vi "test_read-nmea-data2.vi"() -> ()   [LabVIEW 2019] (continued)
F9P\t$GBGSV,2,1,06,07,,,23,11,48,133,26,14,87,101,29,28,,,23,1*76\n\t\n15:15:02.67\tF9P\t$GBGSV,2,2,06,33,62,220,31,34,,,25,1*46\n\t\n15:15:02.69\tF9P\t$GBGSV,1,1,03,11,48,133,,14,87,101,28,33,62,220,,3*4E\n\t\n15:15:02.71\tF9P\t$GNGLL,3723.60146,N,12656.95282,E,061504.00,A,A*73\n\t\n15:15:02.73\tF9P\t\t\n15:15:02.75\tF9P\t\t\n15:15:02.77\tF9P\t\t\n15:15:02.79\tF9P\t\t\n15:15:02.81\tF9P\t\t\n15:15:02.83\tF9P\t\t\n15:15:02.85\tF9P\t\t\n15:15:02.87\tF9P\t\t\n15:15:02.89\tF9P\t\t\n15:15:02.91\tF9P\t\t\n15:15:02.93\tF9P\t\t\n15:15:02.95\tF9P\t\t\n15:15:02.97\tF9P\t\t\n15:15:02.99\tF9P\t\t\n15:15:03.02\tF9P\t\t\n15:15:03.04\tF9P\t\t\n15:15:03.06\tF9P\t\t\n15:15:03.08\tF9P\t\t\n15:15:03.10\tF9P\t\t\n15:15:03.12\tF9P\t\t\n15:15:03.14\tF9P\t\t\n15:15:03.16\tF9P\t\t\n15:15:03.18\tF9P\t\t\n15:15:03.20\tF9P\t\t\n15:15:03.22\tF9P\t\t\n15:15:03.24\tF9P\t$GNRMC,061505.00,A,3723.60131,N,12656.95173,E,2.899,253.95,250720,,,A,V*02\n\t\n15:15:03.26\tF9P\t$GNVTG,253.95,T,,M,2.899,N,5.368,K,A*29\n\t\n15:15:03.28\tF9P\t$GNGGA,061505.00,3723.60131,N,12656.95173,E,1,12,0.74,45.5,M,18.5,M,,*72\n\t\n15:15:03.30\tF9P\t$GNGSA,A,3,12,06,19,05,17,09,04,02,,,,,1.25,0.74,1.01,1*05\n\t\n15:15:03.32\tF9P\t$GNGSA,A,3,85,70,71,84,,,,,,,,,1.25,0.74,1.01,2*07\n\t\n15:15:03.34\tF9P\t$GNGSA,A,3,36,19,11,04,09,12,,,,,,,1.25,0.74,1.01,3*05\n\t\n15:15:03.36\tF9P\t$GNGSA,A,3,14,11,33,,,,,,,,,,1.25,0.74,1.01,4*04\n\t\n15:15:03.38\tF9P\t$GPGSV,3,1,09,02,56,320,26,04,17,043,37,05,38,248,39,06,64,051,39,1*6A\n\t\n15:15:03.40\tF9P\t$GPGSV,3,2,09,09,44,072,38,12,23,275,27,17,31,154,31,19,51,157,27,1*60\n\t\n15:15:03.42\tF9P\t$GPGSV,3,3,09,25,12,306,15,1*58\n\t\n15:15:03.44\tF9P\t$GPGSV,3,1,09,02,56,320,,04,17,043,22,05,38,248,27,06,64,051,29,6*63\n\t\n15:15:03.46\tF9P\t$GPGSV,3,2,09,09,44,072,29,12,23,275,18,17,31,154,20,19,51,157,,6*6E\n\t\n15:15:03.48\tF9P\t$GPGSV,3,3,09,25,12,306,,6*5B\n\t\n15:15:03.50\tF9P\t$GLGSV,2,1,08,69,10,031,26,70,70,037,29,71,54,207,35,72,05,210,,1*73\n\t\n15:15:03.52\tF9P\t$GLGSV,2,2,08,77,01,324,,84,19,123,17,85,69,072,25,86,38,331,,1*72\n\t\n15:15:03.54\tF9P\t$GLGSV,2,1,08,69,10,031,18,70,70,037,,71,54,207,25,72,05,210,,3*76\n\t\n15:15:03.56\tF9P\t$GLGSV,2,2,08,77,01,324,,84,19,123,22,85,69,072,27,86,38,331,,3*74\n\t\n15:15:03.58\tF9P\t$GAGSV,2,1,08,02,08,296,10,04,67,115,37,09,33,193,26,11,72,001,24,7*7E\n\t\n15:15:03.60\tF9P\t$GAGSV,2,2,08,12,39,103,31,19,25,045,33,25,08,248,,36,27,309,22,7*77\n\t\n15:15:03.62\tF9P\t$GAGSV,2,1,08,02,08,296,,04,67,115,,09,33,193,,11,72,001,,2*7C\n\t\n15:15:03.64\tF9P\t$GAGSV,2,2,08,12,39,103,,19,25,045,23,25,08,248,,36,27,309,,2*71\n\t\n15:15:03.66\tF9P\t$GBGSV,2,1,06,07,,,21,11,48,133,26,14,87,101,22,28,,,23,1*7F\n\t\n15:15:03.68\tF9P\t$GBGSV,2,2,06,33,62,220,30,34,,,25,1*47\n\t\n15:15:03.70\tF9P\t$GBGSV,1,1,03,11,48,133,,14,87,101,28,33,62,220,,3*4E\n\t\n15:15:03.72\tF9P\t$GNGLL,3723.60131,N,12656.95173,E,061505.00,A,A*7F\n\t\n15:15:03.74\tF9P\t\t\n15:15:03.76\tF9P\t\t\n15:15:03.78\tF9P\t\t\n15:15:03.80\tF9P\t\t\n15:15:03.82\tF9P\t\t\n15:15:03.84\tF9P\t\t\n15:15:03.86\tF9P\t\t\n15:15:03.88\tF9P\t\t\n15:15:03.90\tF9P\t\t\n15:15:03.92\tF9P\t\t\n15:15:03.94\tF9P\t\t\n15:15:03.96\tF9P\t\t\n15:15:03.98\tF9P\t\t\n15:15:04.00\tF9P\t\t\n15:15:04.02\tF9P\t\t\n15:15:04.04\tF9P\t\t\n15:15:04.06\tF9P\t\t\n15:15:04.08\tF9P\t\t\n15:15:04.10\tF9P\t\t\n15:15:04.12\tF9P\t\t\n15:15:04.14\tF9P\t\t\n15:15:04.16\tF9P\t\t\n15:15:04.18\tF9P\t\t\n15:15:04.20\tF9P\t\t\n15:15:04.22\tF9P\t\t\n15:15:04.24\tF9P\t$GNRMC,061506.00,A,3723.60131,N,12656.95050,E,2.846,256.78,250720,,,A,V*05\n\t\n15:15:04.26\tF9P\t$GNVTG,256.78,T,,M,2.846,N,5.272,K,A*27\n\t\n15:15:04.28\tF9P\t$GNGGA,061506.00,3723.60131,N,12656.95050,E,1,12,0.74,45.5,M,18.5,M,,*71\n\t\n15:15:04.30\tF9P\t$GNGSA,A,3,12,06,19,05,17,09,04,02,,,,,1.25,0.74,1.01,1*05\n\t\n15:15:04.32\tF9P\t$GNGSA,A,3,85,70,71,84,,,,,,,,,1.25,0.74,1.01,2*07\n\t\n15:15:04.34\tF9P\t$GNGSA,A,3,36,19,11,04,09,12,,,,,,,1.25,0.74,1.01,3*05\n\t\n15:15:04.36\tF9P\t$GNGSA,A,3,14,11,33,,,,,,,,,,1.25,0.74,1.01,4*04\n\t\n15:15:04.38\tF9P\t$GPGSV,3,1,09,02,56,320,27,04,17,043,35,05,38,248,37,06,64,051,39,1*67\n\t\n15:15:04.40\tF9P\t$GPGSV,3,2,09,09,44,072,38,12,23,275,27,17,31,154,30,19,51,157,28,1*6E\n\t\n15:15:04.42\tF9P\t$GPGSV,3,3,09,25,12,306,15,1*58\n\t\n15:15:04.44\tF9P\t$GPGSV,3,1,09,02,56,320,,04,17,043,21,05,38,248,27,06,64,051,30,6*68\n\t\n15:15:04.46\tF9P\t$GPGSV,3,2,09,09,44,072,29,12,23,275,21,17,31,154,20,19,51,157,,6*64\n\t\n15:15:04.48\tF9P\t$GPGSV,3,3,09,25,12,306,,6*5B\n\t\n15:15:04.50\tF9P\t$GLGSV,2,1,08,69,10,031,32,70,70,037,27,71,54,207,37,72,05,210,,1*7A\n\t\n15:15:04.52\tF9P\t$GLGSV,2,2,08,77,01,324,,84,19,123,15,85,69,072,32,86,38,331,,1*76\n\t\n15:15:04.54\tF9P\t$GLGSV,2,1,08,69,10,031,19,70,70,037,,71,54,207,30,72,05,210,,3*73\n\t\n15:15:04.56\tF9P\t$GLGSV,2,2,08,77,01,324,,84,19,123,23,85,69,072,31,86,38,331,,3*72\n\t\n15:15:04.58\tF9P\t$GAGSV,2,1,08,02,08,296,07,04,67,115,31,09,33,193,31,11,72,001,23,7*7F\n\t\n15:15:04.60\tF9P\t$GAGSV,2,2,08,12,39,103,25,19,25,045,33,25,08,248,,36,27,309,21,7*71\n\t\n15:15:04.62\tF9P\t$GAGSV,2,1,08,02,08,296,,04,67,115,,09,33,193,,11,72,001,,2*7C\n\t\n15:15:04.64\tF9P\t$GAGSV,2,2,08,12,39,103,,19,25,045,23,25,08,248,,36,27,309,,2*71\n\t\n15:15:04.66\tF9P\t$GBGSV,2,1,06,07,,,19,11,48,133,26,14,87,101,30,28,,,23,1*77\n\t\n15:15:04.68\tF9P\t$GBGSV,2,2,06,33,62,220,33,34,,,32,1*42\n\t\n15:15:04.70\tF9P\t$GBGSV,1,1,03,11,48,133,,14,87,101,28,33,62,220,,3*4E\n\t\n15:15:04.72\tF9P\t$GNGLL,3723.60131,N,12656.95050,E,061506.00,A,A*7C\n\t\n15:15:04.74\tF9P\t\t\n15:15:04.76\tF9P\t\t\n15:15:04.78\tF9P\t\t\n15:15:04.80\tF9P\t\t\n15:15:04.82\tF9P\t\t\n15:15:04.84\tF9P\t\t\n15:15:04.86\tF9P\t\t\n15:15:04.88\tF9P\t\t\n15:15:04.90\tF9P\t\t\n15:15:04.92\tF9P\t\t\n15:15:04.94\tF9P\t\t\n15:15:04.96\tF9P\t\t\n15:15:04.98\tF9P\t\t\n15:15:05.00\tF9P\t\t\n15:15:05.02\tF9P\t\t\n15:15:05.04\tF9P\t\t\n15:15:05.06\tF9P\t\t\n15:15:05.08\tF9P\t\t\n15:15:05.10\tF9P\t\t\n15:15:05.12\tF9P\t\t\n15:15:05.14\tF9P\t\t\n15:15:05.16\tF9P\t\t\n15:15:05.18\tF9P\t\t\n15:15:05.20\tF9P\t\t\n15:15:05.22\tF9P\t\t\n15:15:05.24\tF9P\t$GNRMC,061507.00,A,3723.60139,N,12656.94935,E,2.684,262.17,250720,,,A,V*09\n\t\n15:15:05.26\tF9P\t$GNVTG,262.17,T,,M,2.684,N,4.971,K,A*20\n\t\n15:15:05.28\tF9P\t$GNGGA,061507.00,3723.60139,N,12656.94935,E,1,12,0.74,45.4,M,18.5,M,,*72\n\t\n15:15:05.30\tF9P\t$GNGSA,A,3,12,06,19,05,17,09,04,02,,,,,1.25,0.74,1.01,1*05\n\t\n15:15:05.32\tF9P\t$GNGSA,A,3,85,70,71,84,,,,,,,,,1.25,0.74,1.01,2*07\n\t\n15:15:05.34\tF9P\t$GNGSA,A,3,36,19,11,04,09,12,,,,,,,1.25,0.74,1.01,3*05\n\t\n15:15:05.36\tF9P\t$GNGSA,A,3,14,11,33,,,,,,,,,,1.25,0.74,1.01,4*04\n\t\n15:15:05.38\tF9P\t$GPGSV,3,1,09,02,56,320,32,04,17,043,34,05,38,248,36,06,64,051,38,1*62\n\t\n15:15:05.40\tF9P\t$GPGSV,3,2,09,09,44,072,39,12,23,275,27,17,31,154,29,19,51,157,28,1*67\n\t\n15:15:05.42\tF9P\t$GPGSV,3,3,09,25,12,306,15,1*58\n\t\n15:15:05.44\tF9P\t$GPGSV,3,1,09,02,56,320,,04,17,043,20,05,38,248,29,06,64,051,28,6*6E\n\t\n15:15:05.46\tF9P\t$GPGSV,3,2,09,09,44,072,29,12,23,275,23,17,31,154,18,19,51,157,,6*6D\n\t\n15:15:05.48\tF9P\t$GPGSV,3,3,09,25,12,306,,6*5B\n\t\n15:15:05.50\tF9P\t$GLGSV,2,1,08,69,10,031,31,70,70,037,27,71,54,207,37,72,05,210,,1*79\n\t\n15:15:05.52\tF9P\t$GLGSV,2,2,08,77,01,324,,84,19,123,16,85,69,072,29,86,38,331,,1*7F\n\t\n15:15:05.54\tF9P\t$GLGSV,2,1,08,69,10,031,20,70,70,037,,71,54,207,26,72,05,210,,3*7E\n\t\n15:15:05.56\tF9P\t$GLGSV,2,2,08,77,01,324,,84,19,123,23,85,69,072,24,86,38,331,,3*76\n\t\n15:15:05.58\tF9P\t$GAGSV,2,1,08,02,08,296,11,04,67,115,38,09,33,193,25,11,72,001,23,7*74\n\t\n15:15:05.60\tF9P\t$GAGSV,2,2,08,12,39,103,26,19,25,045,28,25,08,248,,36,27,309,21,7*78\n\t\n15:15:05.62\tF9P\t$GAGSV,2,1,08,02,08,296,,04,67,115,,09,33,193,,11,72,001,,2*7C\n\t\n15:15:05.64\tF9P\t$GAGSV,2,2,08,12,39,103,,19,25,045,22,25,08,248,,36,27,309,,2*70\n\t\n15:15:05.66\tF9P\t$GBGSV,2,1,06,07,,,22,11,48,133,26,14,87,101,23,28,,,24,1*7A\n\t\n15:15:05.68\tF9P\t$GBGSV,2,2,06,33,62,220,28,34,,,27,1*4C\n\t\n15:15:05.70\tF9P\t$GBGSV,1,1,03,11,48,133,,14,87,101,27,33,62,220,,3*41\n\t\n15:15:05.72\tF9P\t$GNGLL,3723.60139,N,12656.94935,E,061507.00,A,A*7E\n\t\n15:15:05.74\tF9P\t\t\n15:15:05.76\tF9P\t\t\n15:15:05.78\tF9P\t\t\n15:15:05.80\tF9P\t\t\n15:15:05.82\tF9P\t\t\n15:15:05.84\tF9P\t\t\n15:15:05.86\tF9P\t\t\n15:15:05.88\tF9P\t\t\n15:15:05.90\tF9P\t\t\n15:15:05.92\tF9P\t\t\n15:15:05.94\tF9P\t\t\n15:15:05.96\tF9P\t\t\n15:15:05.98\tF9P\t\t\n15:15:06.00\tF9P\t\t\n15:15:06.02\tF9P\t\t\n15:15:06.04\tF9P\t\t\n15:15:06.06\tF9P\t\t\n15:15:06.08\tF9P\t\t\n15:15:06.10\tF9P\t\t\n15:15:06.12\tF9P\t\t\n15:15:06.14\tF9P\t\t\n15:15:06.16\tF9P\t\t\n15:15:06.18\tF9P\t\t\n15:15:06.20\tF9P\t\t\n15:15:06.22\tF9P\t\t\n15:15:06.24\tF9P\t$GNRMC,061508.00,A,3723.60141,N,12656.94831,E,2.548,261.80,250720,,,A,V*02\n\t\n15:15:06.26\tF9P\t$GNVTG,261.80,T,,M,2.548,N,4.719,K,A*2E\n\t\n15:15:06.28\tF9P\t$GNGGA,061508.00,3723.60141,N,12656.94831,E,1,12,0.72,45.4,M,18.5,M,,*71\n\t\n15:15:06.30\tF9P\t$GNGSA,A,3,12,06,19,05,17,09,04,02,,,,,1.23,0.72,1.00,1*04\n\t\n15:15:06.32\tF9P\t$GNGSA,A,3,85,70,71,84,,,,,,,,,1.23,0.72,1.00,2*06\n\t\n15:15:06.34\tF9P\t$GNGSA,A,3,36,19,11,04,09,12,,,,,,,1.23,0.72,1.00,3*04\n\t\n15:15:06.36\tF9P\t$GNGSA,A,3,14,11,33,,,,,,,,,,1.23,0.72,1.00,4*05\n\t\n15:15:06.38\tF9P\t$GPGSV,3,1,09,02,56,320,25,04,17,043,37,05,38,248,36,06,64,051,37,1*68\n\t\n15:15:06.40\tF9P\t$GPGSV,3,2,09,09,44,072,42,12,23,275,27,17,31,154,25,19,51,157,29,1*66\n\t\n15:15:06.42\tF9P\t$GPGSV,3,3,09,25,12,305,15,1*5B\n\t\n15:15:06.44\tF9P\t$GPGSV,3,1,09,02,56,320,,04,17,043,19,05,38,248,28,06,64,051,30,6*6C\n\t\n15:15:06.46\tF9P\t$GPGSV,3,2,09,09,44,072,30,12,23,275,22,17,31,154,18,19,51,157,,6*64\n\t\n15:15:06.48\tF9P\t$GPGSV,3,3,09,25,12,305,,6*58\n\t\n15:15:06.50\tF9P\t$GLGSV,2,1,08,69,10,031,28,70,70,037,26,71,54,207,34,72,05,210,,1*73\n\t\n15:15:06.52\tF9P\t$GLGSV,2,2,08,77,01,324,,84,19,123,16,85,69,072,25,86,38,331,,1*73\n\t\n15:15:06.54\tF9P\t$GLGSV,2,1,08,69,10,031,22,70,70,037,,71,54,207,25,72,05,210,,3*7F\n\t\n15:15:06.56\tF9P\t$GLGSV,2,2,08,77,01,324,,84,19,123,21,85,69,072,31,86,38,331,,3*70\n\t\n15:15:06.58\tF9P\t$GAGSV,2,1,08,02,08,296,11,04,67,115,38,09,33,193,25,11,72,001,28,7*7F\n\t\n15:15:06.60\tF9P\t$GAGSV,2,2,08,12,39,103,26,19,25,045,23,25,08,248,,36,27,309,22,7*70\n\t\n15:15:06.62\tF9P\t$GAGSV,2,1,08,02,08,296,,04,67,115,,09,33,193,,11,72,001,,2*7C\n\t\n15:15:06.64\tF9P\t$GAGSV,2,2,08,12,39,103,,19,25,045,21,25,08,248,,36,27,309,,2*73\n\t\n15:15:06.66\tF9P\t$GBGSV,2,1,06,07,,,24,11,48,133,27,14,87,101,30,28,,,23,1*78\n\t\n15:15:06.68\tF9P\t$GBGSV,2,2,06,33,62,220,28,34,,,27,1*4C\n\t\n15:15:06.70\tF9P\t$GBGSV,1,1,03,11,48,133,,14,87,101,27,33,62,220,,3*41\n\t\n15:15:06.72\tF9P\t$GNGLL,3723.60141,N,12656.94831,E,061508.00,A,A*7B\n\t\n15:15:06.74\tF9P\t\t\n15:15:06.76\tF9P\t\t\n15:15:06.78\tF9P\t\t\n15:15:06.80\tF9P\t\t\n15:15:06.82\tF9P\t\t\n15:15:06.84\tF9P\t\t\n15:15:06.86\tF9P\t\t\n15:15:06.88\tF9P\t\t\n15:15:06.90\tF9P\t\t\n15:15:06.92\tF9P\t\t\n15:15:06.94\tF9P\t\t\n15:15:06.96\tF9P\t\t\n15:15:06.98\tF9P\t\t\n15:15:07.00\tF9P\t\t\n15:15:07.02\tF9P\t\t\n15:15:07.04\tF9P\t\t\n15:15:07.06\tF9P\t\t\n15:15:07.08\tF9P\t\t\n15:15:07.10\tF9P\t\t\n15:15:07.12\tF9P\t\t\n15:15:07.14\tF9P\t\t\n15:15:07.16\tF9P\t\t\n15:15:07.18\tF9P\t\t\n15:15:07.20\tF9P\t\t\n15:15:07.22\tF9P\t\t\n15:15:07.24\tF9P\t$GNRMC,061509.00,A,3723.60129,N,12656.94727,E,2.766,257.31,250720,,,A,V*04\n\t\n15:15:07.26\tF9P\t$GNVTG,257.31,T,,M,2.766,N,5.122,K,A*20\n\t\n15:15:07.28\tF9P\t$GNGGA,061509.00,3723.60129,N,12656.94727,E,1,12,0.76,45.1,M,18.5,M,,*77\n\t\n15:15:07.30\tF9P\t$GNGSA,A,3,12,06,19,05,17,09,04,02,,,,,1.28,0.76,1.03,1*08\n\t\n15:15:07.32\tF9P\t$GNGSA,A,3,85,70,71,84,,,,,,,,,1.28,0.76,1.03,2*0A\n\t\n15:15:07.34\tF9P\t$GNGSA,A,3,36,19,11,04,09,12,,,,,,,1.28,0.76,1.03,3*08\n\t\n15:15:07.36\tF9P\t$GNGSA,A,3,14,11,33,,,,,,,,,,1.28,0.76,1.03,4*09\n\t\n15:15:07.38\tF9P\t$GPGSV,3,1,09,02,56,320,25,04,17,043,39,05,38,248,37,06,64,051,37,1*67\n\t\n15:15:07.40\tF9P\t$GPGSV,3,2,09,09,44,072,35,12,23,275,26,17,31,154,30,19,51,157,28,1*62\n\t\n15:15:07.42\tF9P\t$GPGSV,3,3,09,25,12,305,14,1*5A\n\t\n15:15:07.44\tF9P\t$GPGSV,3,1,09,02,56,320,,04,17,043,18,05,38,248,28,06,64,051,31,6*6C\n\t\n15:15:07.46\tF9P\t$GPGSV,3,2,09,09,44,072,30,12,23,275,22,17,31,154,17,19,51,157,,6*6B\n\t\n15:15:07.48\tF9P\t$GPGSV,3,3,09,25,12,305,,6*58\n\t\n15:15:07.50\tF9P\t$GLGSV,2,1,08,69,10,031,33,70,70,037,28,71,54,207,36,72,05,210,,1*75\n\t\n15:15:07.52\tF9P\t$GLGSV,2,2,08,77,01,324,,84,19,123,16,85,69,072,34,86,38,331,,1*73\n\t\n15:15:07.54\tF9P\t$GLGSV,2,1,08,69,10,031,20,70,70,037,,71,54,207,30,72,05,210,,3*79\n\t\n15:15:07.56\tF9P\t$GLGSV,2,2,08,77,01,324,,84,19,123,20,85,69,072,31,86,38,331,,3*71\n\t\n15:15:07.58\tF9P\t$GAGSV,2,1,08,02,08,296,09,04,67,115,32,09,33,193,24,11,72,001,26,7*73\n\t\n15:15:07.60\tF9P\t$GAGSV,2,2,08,12,39,103,26,19,25,045,34,25,08,248,,36,27,309,22,7*76\n\t\n15:15:07.62\tF9P\t$GAGSV,2,1,08,02,08,296,,04,67,115,,09,33,193,,11,72,001,,2*7C\n\t\n15:15:07.64\tF9P\t$GAGSV,2,2,08,12,39,103,,19,25,045,22,25,08,248,,36,27,309,,2*70\n\t\n15:15:07.66\tF9P\t$GBGSV,2,1,06,07,,,22,11,48,133,26,14,87,101,29,28,,,22,1*76\n\t\n15:15:07.68\tF9P\t$GBGSV,2,2,06,33,62,220,30,34,,,31,1*42\n\t\n15:15:07.70\tF9P\t$GBGSV,1,1,03,11,48,133,,14,87,101,27,33,62,220,,3*41\n\t\n15:15:07.72\tF9P\t$GNGLL,3723.60129,N,12656.94727,E,061509.00,A,A*7C\n\t\n15:15:07.74\tF9P\t\t\n15:15:07.76\tF9P\t\t\n15:15:07.78\tF9P\t\t\n15:15:07.80\tF9P\t\t\n15:15:07.82\tF9P\t\t\n15:15:07.84\tF9P\t\t\n15:15:07.86\tF9P\t\t\n15:15:07.88\tF9P\t\t\n15:15:07.90\tF9P\t\t\n15:15:07.92\tF9P\t\t\n15:15:07.94\tF9P\t\t\n15:15:07.96\tF9P\t\t\n15:15:07.98\tF9P\t\t\n15:15:08.00\tF9P\t\t\n15:15:08.02\tF9P\t\t\n15:15:08.04\tF9P\t\t\n15:15:08.06\tF9P\t\t\n15:15:08.08\tF9P\t\t\n15:15:08.10\tF9P\t\t\n15:15:08.12\tF9P\t\t\n15:15:08.14\tF9P\t\t\n15:15:08.16\tF9P\t\t\n15:15:08.18\tF9P\t\t\n15:15:08.20\tF9P\t\t\n15:15:08.22\tF9P\t\t\n15:15:08.24\tF9P\t$GNRMC,061510.00,A,3723.60114,N,12656.94617,E,2.826,256.05,250720,,,A,V*0D\n\t\n15:15:08.26\tF9P\t$GNVTG,256.05,T,,M,2.826,N,5.234,K,A*29\n\t\n15:15:08.28\tF9P\t$GNGGA,061510.00,3723.60114,N,12656.94617,E,1,12,0.76,45.0,M,18.5,M,,*72\n\t\n15:15:08.30\tF9P\t$GNGSA,A,3,12,06,19,05,17,09,04,02,,,,,1.28,0.76,1.03,1*08\n\t\n15:15:08.32\tF9P\t$GNGSA,A,3,85,70,71,84,,,,,,,,,1.28,0.76,1.03,2*0A\n\t\n15:15:08.34\tF9P\t$GNGSA,A,3,36,19,11,04,09,12,,,,,,,1.28,0.76,1.03,3*08\n\t\n15:15:08.36\tF9P\t$GNGSA,A,3,14,11,33,,,,,,,,,,1.28,0.76,1.03,4*09\n\t\n15:15:08.38\tF9P\t$GPGSV,3,1,09,02,56,320,25,04,17,043,30,05,38,248,38,06,64,051,38,1*6E\n\t\n15:15:08.40\tF9P\t$GPGSV,3,2,09,09,44,072,27,12,23,275,32,17,31,154,31,19,51,157,27,1*6A\n\t\n15:15:08.42\tF9P\t$GPGSV,3,3,09,25,12,305,12,1*5C\n\t\n15:15:08.44\tF9P\t$GPGSV,3,1,09,02,56,320,,04,17,043,19,05,38,248,29,06,64,051,31,6*6C\n\t\n15:15:08.46\tF9P\t$GPGSV,3,2,09,09,44,072,30,12,23,275,19,17,31,154,19,19,51,157,,6*6D\n\t\n15:15:08.48\tF9P\t$GPGSV,3,3,09,25,12,305,,6*58\n\t\n15:15:08.50\tF9P\t$GLGSV,2,1,08,69,10,031,25,70,70,037,28,71,54,207,41,72,05,210,,1*72\n\t\n15:15:08.52\tF9P\t$GLGSV,2,2,08,77,01,324,,84,19,123,16,85,69,072,26,86,38,331,,1*70\n\t\n15:15:08.54\tF9P\t$GLGSV,2,1,08,69,10,031,18,70,70,037,,71,54,207,23,72,05,210,,3*70\n\t\n15:15:08.56\tF9P\t$GLGSV,2,2,08,77,01,324,,84,19,123,18,85,69,072,32,86,38,331,,3*79\n\t\n15:15:08.58\tF9P\t$GAGSV,2,1,08,02,08,296,12,04,67,115,34,09,33,193,23,11,72,001,24,7*7A\n\t\n15:15:08.60\tF9P\t$GAGSV,2,2,08,12,39,103,25,19,25,045,29,25,08,248,,36,27,309,22,7*79\n\t\n15:15:08.62\tF9P\t$GAGSV,2,1,08,02,08,296,,04,67,115,,09,33,193,,11,72,001,,2*7C\n\t\n15:15:08.64\tF9P\t$GAGSV,2,2,08,12,39,103,,19,25,045,22,25,08,248,,36,27,309,,2*70\n\t\n15:15:08.66\tF9P\t$GBGSV,2,1,06,07,,,21,11,48,133,28,14,87,101,20,28,,,22,1*72\n\t\n15:15:08.68\tF9P\t$GBGSV,2,2,06,33,62,220,30,34,,,29,1*4B\n\t\n15:15:08.70\tF9P\t$GBGSV,1,1,03,11,48,133,,14,87,101,30,33,62,220,,3*47\n\t\n15:15:08.72\tF9P\t$GNGLL,3723.60114,N,12656.94617,E,061510.00,A,A*78\n\t\n15:15:08.74\tF9P\t\t\n15:15:08.76\tF9P\t\t\n15:15:08.78\tF9P\t\t\n15:15:08.80\tF9P\t\t\n15:15:08.82\tF9P\t\t\n15:15:08.84\tF9P\t\t\n15:15:08.86\tF9P\t\t\n15:15:08.88\tF9P\t\t\n15:15:08.90\tF9P\t\t\n15:15:08.92\tF9P\t\t\n15:15:08.94\tF9P\t\t\n15:15:08.96\tF9P\t\t\n15:15:08.98\tF9P\t\t\n15:15:09.00\tF9P\t\t\n15:15:09.02\tF9P\t\t\n15:15:09.04\tF9P\t\t\n15:15:09.06\tF9P\t\t\n15:15:09.08\tF9P\t\t\n15:15:09.10\tF9P\t\t\n15:15:09.12\tF9P\t\t\n15:15:09.14\tF9P\t\t\n15:15:09.16\tF9P\t\t\n15:15:09.18\tF9P\t\t\n15:15:09.20\tF9P\t\t\n15:15:09.22\tF9P\t$GNRMC,061511.00,A,3723.60102,N,12656.94524,E,2.590,256.42,250720,,,A,V*0B\n\t\n15:15:09.24\tF9P\t$GNVTG,256.42,T,,M,2.590,N,4.796,K,A*26\n\t\n15:15:09.26\tF9P\t$GNGGA,061511.00,3723.60102,N,12656.94524,E,1,12,0.72,45.1,M,18.5,M,,*72\n\t\n15:15:09.28\tF9P\t$GNGSA,A,3,12,06,19,05,17,09,04,02,,,,,1.23,0.72,1.00,1*04\n\t\n15:15:09.30\tF9P\t$GNGSA,A,3,85,70,71,84,,,,,,,,,1.23,0.72,1.00,2*06\n\t\n15:15:09.32\tF9P\t$GNGSA,A,3,36,19,11,04,09,12,,,,,,,1.23,0.72,1.00,3*04\n\t\n15:15:09.34\tF9P\t$GNGSA,A,3,14,11,33,,,,,,,,,,1.23,0.72,1.00,4*05\n\t\n15:15:09.36\tF9P\t$GPGSV,3,1,09,02,56,320,26,04,17,043,30,05,38,248,32,06,64,051,39,1*66\n\t\n15:15:09.38\tF9P\t$GPGSV,3,2,09,09,44,072,39,12,23,275,27,17,31,154,31,19,51,157,27,1*61\n\t\n15:15:09.40\tF9P\t$GPGSV,3,3,09,25,12,305,09,1*56\n\t\n15:15:09.42\tF9P\t$GPGSV,3,1,09,02,56,320,,04,17,043,21,05,38,248,22,06,64,051,26,6*6A\n\t\n15:15:09.44\tF9P\t$GPGSV,3,2,09,09,44,072,33,12,23,275,20,17,31,154,19,19,51,157,,6*64\n\t\n15:15:09.46\tF9P\t$GPGSV,3,3,09,25,12,305,,6*58\n\t\n15:15:09.48\tF9P\t$GLGSV,2,1,08,69,10,031,26,70,70,037,28,71,54,207,40,72,05,210,,1*70\n\t\n15:15:09.50\tF9P\t$GLGSV,2,2,08,77,01,324,,84,19,123,17,85,69,072,25,86,38,331,,1*72\n\t\n15:15:09.52\tF9P\t$GLGSV,2,1,08,69,10,031,18,70,70,037,,71,54,207,30,72,05,210,,3*72\n\t\n15:15:09.54\tF9P\t$GLGSV,2,2,08,77,01,324,,84,19,123,18,85,69,072,26,86,38,331,,3*7C\n\t\n15:15:09.56\tF9P\t$GAGSV,2,1,08,02,08,296,12,04,67,115,32,09,33,193,23,11,72,001,25,7*7D\n\t\n15:15:09.58\tF9P\t$GAGSV,2,2,08,12,39,103,23,19,25,045,28,25,08,248,,36,27,309,21,7*7D\n\t\n15:15:09.60\tF9P\t$GAGSV,2,1,08,02,08,296,,04,67,115,,09,33,193,,11,72,001,,2*7C\n\t\n15:15:09.63\tF9P\t$GAGSV,2,2,08,12,39,103,,19,25,045,21,25,08,248,,36,27,309,,2*73\n\t\n15:15:09.65\tF9P\t$GBGSV,2,1,06,07,,,19,11,48,133,28,14,87,101,33,28,,,23,1*7A\n\t\n15:15:09.67\tF9P\t$GBGSV,2,2,06,33,62,220,27,34,,,19,1*4E\n\t\n15:15:09.69\tF9P\t$GBGSV,1,1,03,11,48,133,,14,87,101,,33,62,220,,3*44\n\t\n15:15:09.71\tF9P\t$GNGLL,3723.60102,N,12656.94524,E,061511.00,A,A*7D\n\t\n15:15:09.73\tF9P\t\t\n15:15:09.75\tF9P\t\t\n15:15:09.77\tF9P\t\t\n15:15:09.79\tF9P\t\t\n15:15:09.81\tF9P\t\t\n15:15:09.83\tF9P\t\t\n15:15:09.85\tF9P\t\t\n15:15:09.87\tF9P\t\t\n15:15:09.89\tF9P\t\t\n15:15:09.91\tF9P\t\t\n15:15:09.93\tF9P\t\t\n15:15:09.95\tF9P\t\t\n15:15:09.97\tF9P\t\t\n15:15:09.99\tF9P\t\t\n15:15:10.01\tF9P\t\t\n15:15:10.03\tF9P\t\t\n15:15:10.05\tF9P\t\t\n15:15:10.07\tF9P\t\t\n15:15:10.09\tF9P\t\t\n15:15:10.11\tF9P\t\t\n15:15:10.13\tF9P\t\t\n15:15:10.15\tF9P\t\t\n15:15:10.17\tF9P\t\t\n15:15:10.19\tF9P\t\t\n15:15:10.21\tF9P\t\t\n15:15:10.23\tF9P\t\t\n15:15:10.25\tF9P\t$GNRMC,061512.00,A,3723.60078,N,12656.94421,E,2.788,253.72,250720,,,A,V*0D\n\t\n15:15:10.27\tF9P\t$GNVTG,253.72,T,,M,2.788,N,5.163,K,A*26\n\t\n15:15:10.29\tF9P\t$GNGGA,061512.00,3723.60078,N,12656.94421,E,1,12,0.79,45.0,M,18.5,M,,*73\n\t\n15:15:10.31\tF9P\t$GNGSA,A,3,12,06,19,05,17,09,04,02,,,,,1.30,0.79,1.03,1*0E\n\t\n15:15:10.33\tF9P\t$GNGSA,A,3,85,70,71,84,,,,,,,,,1.30,0.79,1.03,2*0C\n\t\n15:15:10.35\tF9P\t$GNGSA,A,3,36,19,11,04,09,12,,,,,,,1.30,0.79,1.03,3*0E\n\t\n15:15:10.37\tF9P\t$GNGSA,A,3,14,11,33,,,,,,,,,,1.30,0.79,1.03,4*0F\n\t\n15:15:10.39\tF9P\t$GPGSV,3,1,09,02,56,320,26,04,17,043,31,05,38,248,40,06,64,051,41,1*6D\n\t\n15:15:10.41\tF9P\t$GPGSV,3,2,09,09,44,072,37,12,23,275,26,17,31,154,27,19,51,157,27,1*69\n\t\n15:15:10.43\tF9P\t$GPGSV,3,3,09,25,12,305,08,1*57\n\t\n15:15:10.45\tF9P\t$GPGSV,3,1,09,02,56,320,,04,17,043,19,05,38,
